vi "Send Intake Command.vi"(8 "Wait for Manipulator":bool, 11 "Intake Command":cluster{"Operation":T1, "Outtake":T2}) -> (3 "Is Idle?":bool)   [LabVIEW 2020]
uses:
  intake sub/Implementation/intake sub Operations.ctl
  intake sub/Implementation/Typedef/intake typedef.ctl
  65a954cf-566d-4932-bdc3-28980d65d19b.vi
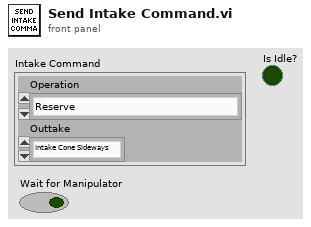
[diagram p1: front panel]
types:
  T1 = typedef "intake sub Operations.ctl" = enum16{"Reserve", "Read Current", "Immediate"}
  T2 = typedef "intake typedef.ctl" = enum16{"Intake Cone Sideways", "Intake Cone Upright", "Intake Cube", "Outtake/Score", "Shoot"}
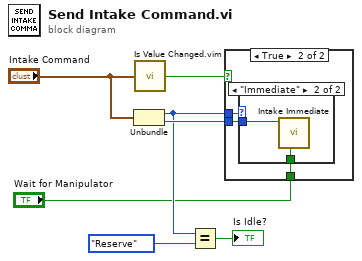
[diagram p0: block diagram]
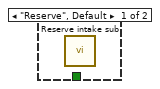
[diagram p3: hidden frame]
diagram:
  n1 = Unbundle("Intake Command") -> ("Operation"=w4:T1, "Outtake"=w6:T2)
  n2 = call "Is Value Changed.vim"("value"="Intake Command") -> ("changed or first call?"=w5:bool)
  n3 = Equal?(x=w4, y=intake_sub_Operations."Reserve") -> (x = y?=→"Is Idle?":bool)
  n4 = case shown="True" w5 {
    tunnel: w4 -> [_ w10]
    tunnel: w6 -> [_ w9]
    tunnel: "Wait for Manipulator" -> [_ w8]
    frame False {
    }
    frame True {
      n5 = case shown="\"Immediate\"" w10 {
        tunnel: w9 -> [_ w12]
        tunnel: w8 -> [_ w11]
        frame "Reserve", Default {
          n6 = call "Reserve intake sub.vi"() -> ()  [unwired: 11 in, 1 out]
        }
        frame "Immediate" {
          n7 = call "Intake Immediate.vi"("Wait for Manipulator"=w11, "intake modes"=w12) -> ()  [unwired: 9 in, 1 out]
        }
      }
    }
  }
